vi "c_ctre_phoenix6_platform_add_schema_string.vi"(0 "String 2":string, 1 "Numeric 2":u16, 2 "String 4":string, 3 "Numeric 3":u32) -> (20 "Numeric":i32, 21 "String":string, 22 "String 3":string)   [LabVIEW 2025]
uses:
  <vilib>/Rock Robotics/WPI/ThirdParty/Phoenix-LabVIEW/Controls/DriverLib.ctl
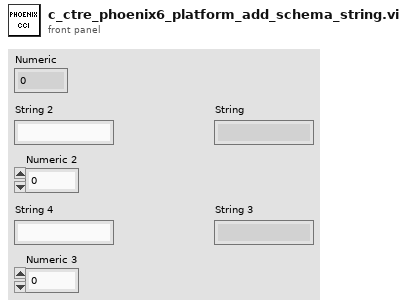
[diagram p1: front panel]
types:
  T1 = typedef "DriverLib.ctl" = path
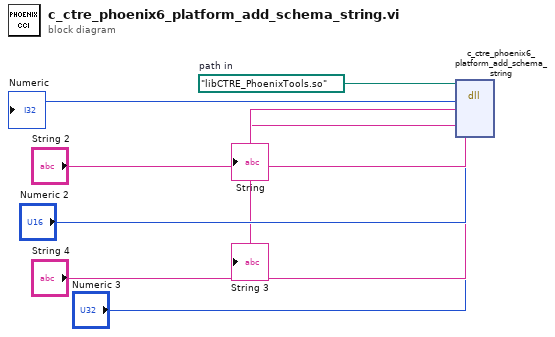
[diagram p0: block diagram]
diagram:
  w8 = T1 path "libCTRE_PhoenixTools.so"  # path in
  n1 = dll-call lib="?" fn="c_ctre_phoenix6_platform_add_schema_string"(path in=w8, "String 2", "Numeric 2", "String 4", "Numeric 3") -> (→"Numeric":i32, →"String":string, →"String 3":string)  [unwired: 4 in, 2 out]
